vi "fgv_AI.vi"(7 "Mode":T1=enum."Update", 8 "error in":errorcluster, 10 "Value":waveform(dbl)[](array[waveform]), 11 "Waveform Graph":refnum<vi>) -> (0 "error out":errorcluster, 1 "mean-vals":dbl[](array[numeric]), 2 "Value 2":waveform(dbl)[](array[waveform]))   [LabVIEW 2019]
uses:
  SubVIs/common/_ctrl/system-status.ctl
  <vilib>/Analysis/baseanly.llb/Mean (DBL).vi
  <vilib>/Analysis/NI_AALBase.lvlib
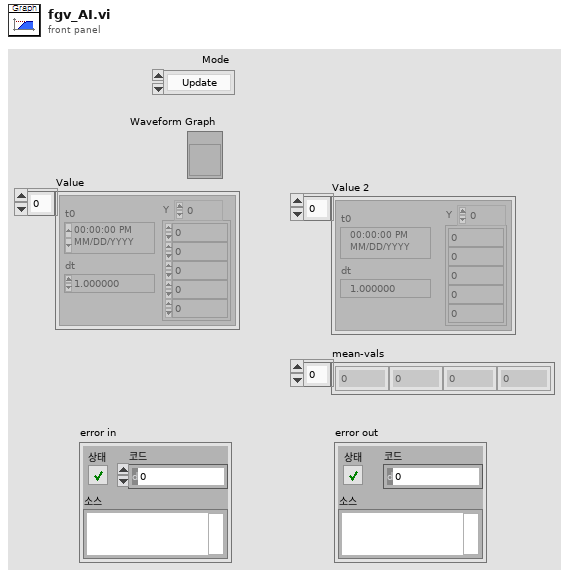
[diagram p1: front panel]
types:
  T1 = typedef "system-status.ctl" = enum16{"Initial", "Update", "Clear", "Read"}
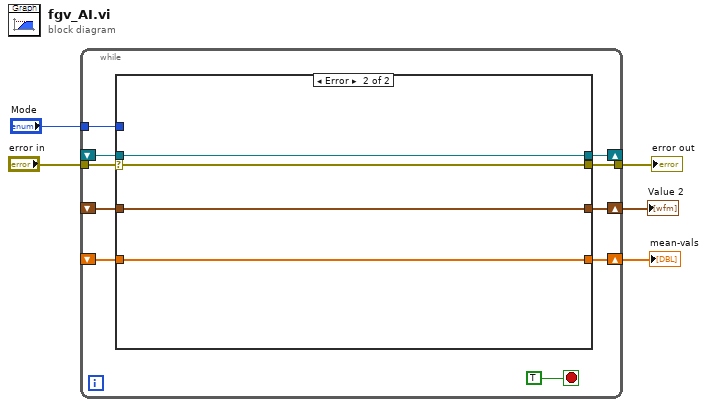
[diagram p0: block diagram]
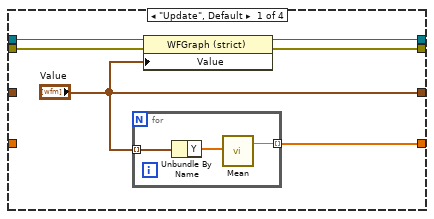
[diagram p3: hidden frame]
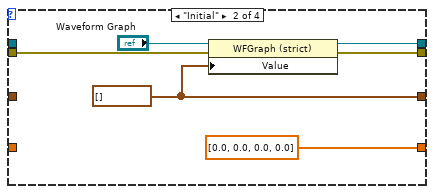
[diagram p4: hidden frame]
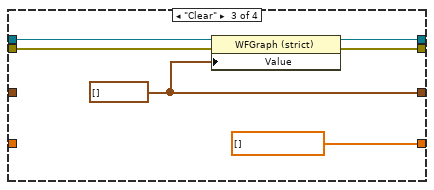
[diagram p5: hidden frame]
diagram:
  n1 = while {
    tunnel: "error in" -> [w10]
    tunnel: [w15] -> w5
    tunnel: "Mode" -> [w13]
    shift-right: [w12] -> _
    shift-left: _ -> [w11]
    shift-right: [w9] -> w2
    shift-left: _ -> [w8]
    shift-right: [w7] -> w1
    shift-left: _ -> [w6]
    stop <- TRUE stop-if-true
    n2 = case shown="Error" w10 {
      selector: w10 -> [w20 w52]
      tunnel: [w24 w52] -> w15
      tunnel: w13 -> [w23 _]
      tunnel: [w22 w53] -> w12
      tunnel: w11 -> [w21 w53]
      tunnel: [w19 w51] -> w9
      tunnel: w8 -> [w18 w51]
      tunnel: [w17 w50] -> w7
      tunnel: w6 -> [w16 w50]
      frame No Error {
        n3 = case shown="\"Read\"" w23 {
          tunnel: w21 -> [w30 _ w43 w48]
          tunnel: w20 -> [w29 w37 w45 w47]
          tunnel: [w27 w38 w44 w47] -> w24
          tunnel: [w28 w39 w42 w48] -> w22
          tunnel: ["Value" w35 w41 w49] -> w19
          tunnel: w18 -> [_ _ _ w49]
          tunnel: [w25 dbl[] [0.0, 0.0, 0.0, 0.0] dbl[] [] w46] -> w17
          tunnel: w16 -> [_ _ _ w46]
          frame "Update", Default {
            n4 = for {
              tunnel: "Value" -> [w33] mode=indexing
              tunnel: [w31] -> w25 mode=indexing
              n5 = Unbundle By Name(w33) -> ("Y"=w32:dbl[])
              n6 = call-poly <vilib>:"Mean.vi"("X"=w32) -> ("mean"=w31:dbl)  [unwired: 1 out]
            }
            n7 = property class="WFGraph (strict)"(reference=w30, error in=w29, "Value"="Value") -> (reference out=w28:refnum<vi>, error out=w27:errorcluster)
          }
          frame "Initial" {
            w35 = waveform(dbl)[] [] ("Value")
            n8 = property class="WFGraph (strict)"(reference="Waveform Graph", error in=w37, "Value"=w35) -> (reference out=w39:refnum<vi>, error out=w38:errorcluster)
          }
          frame "Clear" {
            w41 = waveform(dbl)[] [] ("Value")
            n9 = property class="WFGraph (strict)"(reference=w43, error in=w45, "Value"=w41) -> (reference out=w42:refnum<vi>, error out=w44:errorcluster)
          }
          frame "Read" {
          }
        }
      }
      frame Error {
      }
    }
  }
  "error out" <- w5
  "Value 2" <- w2
  "mean-vals" <- w1
